vi "TI-SigmaGraph.vi"(6 "TI bounds":T4, 7 "sigma/U bounds":T4, 8 "UnderlayPlotSeries":string[](array[string]), 9 "Pre-plot Injection":string, 10 "gnuplotIn":string) -> (2 "gnuplotOut":string)   [LabVIEW 2013]
uses:
  minAndMax.ctl
  AutoManualNumber.ctl
  ticsAndGrids.ctl
  tics.ctl
  grids.ctl
  axisName.ctl
panel:
  in  "CorePlotSeries":string[](array[string])=["FILE index 2 using 1:(jittered($2)) axes x1y1 title 'Turbulence' w points lc rgb '#000080' pt 6 ps 1.5", "FILE index 3 using 1:(jittered($2)) axes x2y1 title 'sigma/U' w points lc rgb '#800000' pt 2 ps 0.8"]
  in  "SigmaTicsAndGrids":T1={"tics"={"ticMin"=0.0, "ticStep"=0.02, "ticMax"=0.1, "minorDivsPerMajor"=2, "ticSpacing"=enum."Auto Tics", "ticPosition"=enum."Outside, no mirror"}, "Grids"={"Gridlines"=enum."No grids", "Zeroaxis"=enum."No zero axis"}, "Mapping"=enum."Lin"}
  in  "TurbulenceTicsAndGrids":T1={"tics"={"ticMin"=0.0, "ticStep"=5.0, "ticMax"=30.0, "minorDivsPerMajor"=2, "ticSpacing"=enum."Auto Tics", "ticPosition"=enum."Outside, no mirror"}, "Grids"={"Gridlines"=enum."Major grid", "Zeroaxis"=enum."No zero axis"}, "Mapping"=enum."Lin"}
  in  "CoreCommand":string="##########################\n# LaTeX markup to modify axis text using previously defined colours \"b\" and \"g\"\nset xtics format '\\color{b}$%g$'\nset x2tics format '\\footnotesize \\color{t}$%g$' offset 0,-0.5\n\nset format y \"\"\t\t\t# Turn off numbers on Y axis\nunset ylabel\t\t\t#  Turn off Y axis label\n\n# Hand-positioned labels, so they can inclue \"point\" command, and using previously defined colours \"b\" and \"g\"\n# X1 label:\nset label '\\color{b}{$Turbulence~Intensity$~(\\%)}' offset 1,-0.2 point lc rgb \"#000080\" pt 6 ps 1.5 at graph 0.15, -0.1\n# X2 label:\nset label '\\footnotesize \\color{t}{$\\sigma(U)/U_{ref}$}' offset 1,-0.2 point lc rgb \"#800000\" pt 2 ps 0.8 at graph 0.35, 1.08\n\nplot \\\n"
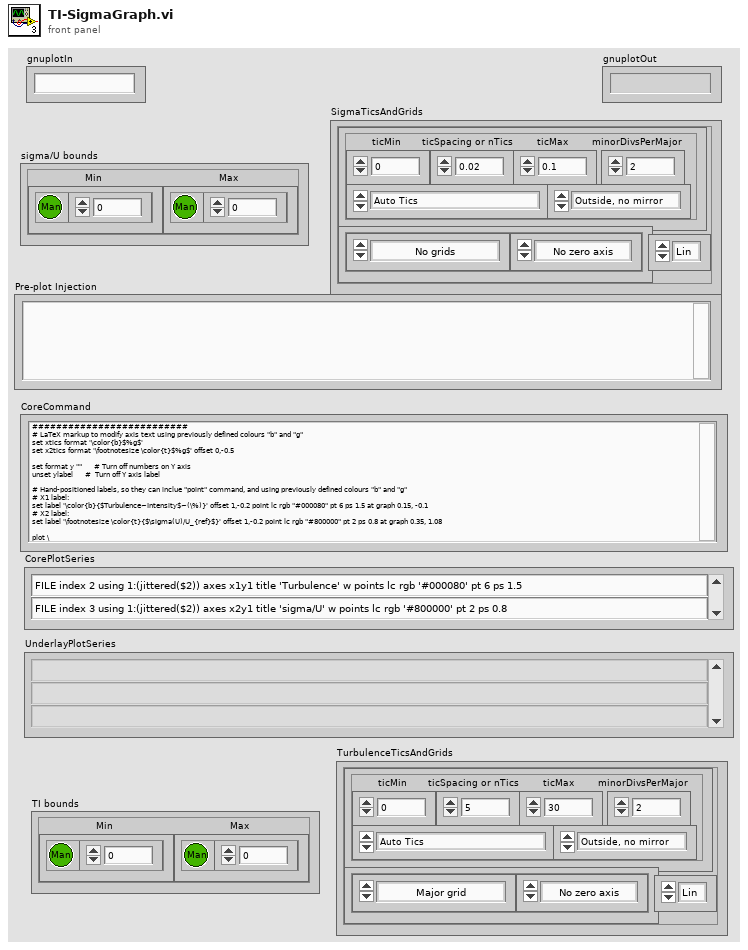
[diagram p1: front panel]
types:
  T1 = typedef "ticsAndGrids.ctl" = cluster{"tics":T2, "Grids":T3, "Mapping":enum8{"Lin", "Log"}}
  T2 = typedef "tics.ctl" = cluster{"ticMin":dbl, "ticStep":dbl, "ticMax":dbl, "minorDivsPerMajor":i32, "ticSpacing":enum16{"Auto Tics", "Fixed spacing", "Fixed Minimum and Spacing", "Start, Spacing and Maximum", "Approx n Tics (rounded)"}, "ticPosition":enum16{"Inside, no mirror", "Inside, mirrored", "Outside, no mirror", "Outside, mirrored", "Invisible"}}
  T3 = typedef "grids.ctl" = cluster{"Gridlines":enum16{"No grids", "Major grid", "Minor grid", "Major and Minor"}, "Zeroaxis":enum16{"No zero axis", "Show zero axis"}}
  T4 = typedef "minAndMax.ctl" = cluster{"Min":T5, "Max":T5}
  T5 = typedef "AutoManualNumber.ctl" = cluster{"Auto":bool, "Value":dbl}
  T6 = typedef "axisName.ctl" = string
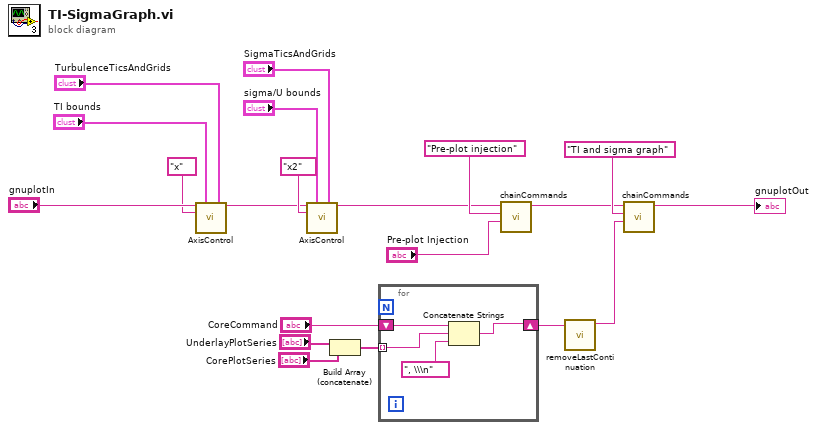
[diagram p0: block diagram]
diagram:
  n1 = call "AxisControl.vi"("String in"="gnuplotIn", "AxisBounds"="TI bounds", "ticsAndGrids"="TurbulenceTicsAndGrids", "Axis"=T6 "x") -> ("String out"=w15:string)  [unwired: 10 in, 1 out]
  n2 = call "AxisControl.vi"("String in"=w15, "AxisBounds"="sigma/U bounds", "ticsAndGrids"="SigmaTicsAndGrids", "Axis"=T6 "x2") -> ("String out"=w2:string)  [unwired: 10 in, 1 out]
  n3 = Build Array (concatenate)("UnderlayPlotSeries", "CorePlotSeries") -> (w9:string[])
  n4 = for {
    tunnel: w9 -> [w24] mode=indexing
    shift-right: [w21] -> w10
    shift-left: "CoreCommand" -> [w22]
    n5 = Concatenate Strings(w22, w24, ", \\\n" ("string")) -> (w21:string)
  }
  n6 = call "chainCommands.vi"("Command"="Pre-plot Injection", "Comments"="Pre-plot injection", "StringIn"=w2) -> ("StringOut"=w1:string)  [unwired: 8 in]
  n7 = call "removeLastContinuation.vi"("String in"=w10) -> ("String out"=w5:string)  [unwired: 10 in]
  n8 = call "chainCommands.vi"("Command"=w5, "Comments"="TI and sigma graph", "StringIn"=w1) -> ("StringOut"=→"gnuplotOut":string)  [unwired: 8 in]
